vi "Start Reading File.vi"(8 "error in (no error)":errorcluster, 10 "TDMS File":path, 11 "TDMS Data Source in":refnum<class "TDMS Data Source.lvclass">) -> (0 "error out":errorcluster, 3 "TDMS Data Source out":refnum<class "TDMS Data Source.lvclass">)   [LabVIEW 2020, in "TDMS Data Source.lvlib" / "TDMS Data Source.lvclass"]
uses:
  TDMS Data Source.lvclass
  QMH Message.ctl
  TDMS Data Source.lvclass/TDMS Data Source.ctl
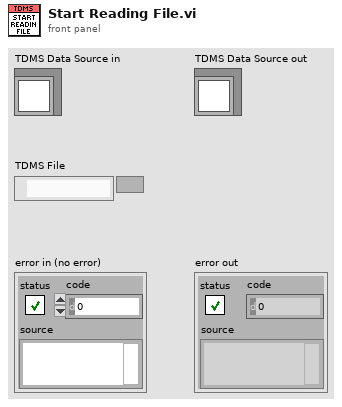
[diagram p1: front panel]
types:
  T1 = typedef "TDMS Data Source.lvlib/TDMS Data Source.lvclass/QMH Message.ctl" = cluster{"Command":string, "Data":variant}
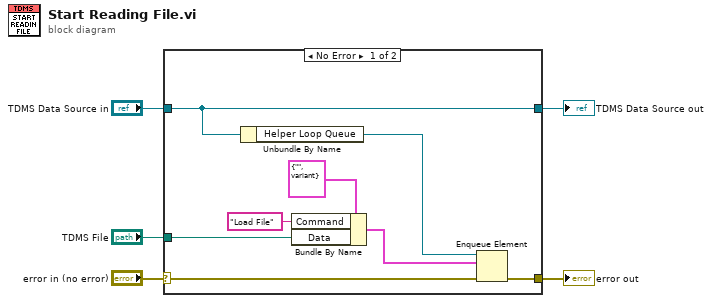
[diagram p0: block diagram]
diagram:
  n1 = case shown="No Error" "error in (no error)" {
    selector: "error in (no error)" -> [w7 w15]
    tunnel: [w6 w15] -> w4
    tunnel: [w13 w14] -> w2
    tunnel: "TDMS Data Source in" -> [w13 w14]
    tunnel: "TDMS File" -> [w10 _]
    frame No Error {
      n2 = Unbundle By Name(w13) -> ("Helper Loop Queue"=w12:refnum<queue>)
      n3 = Bundle By Name(cluster=T1 {"Command"="", "Data"=variant} ("Cluster"), "Command"="Load File", "Data"=w10) -> (w8:T1)
      n4 = Enqueue Element(queue=w12, element=w8, error in (no error)=w7) -> (error out=w6:errorcluster)  [unwired: 1 in, 2 out]
    }
    frame Error {
    }
  }
  "error out" <- w4
  "TDMS Data Source out" <- w2
